vi "bats.parser.test.Single.SequencedUnitHeader.vi"() -> (3 "Passed":bool)   [LabVIEW 2022 SP3]
uses:
  pitch/AddOrder/AddOrderLong.Parameters.ctl
  pitch/ModifyOrder/ModifyOrderLong.Parameters.ctl
  <vilib>/Utility/error.llb/Trim Whitespace One-Sided.vi
  pitch/SequencedUnitHeader/SequencedUnitHeader.lvclass
  pitch/MessageBase/MessageBase.lvclass
  pitch/AddOrder/AddOrderLong.lvclass
  pitch/ModifyOrder/ModifyOrderLong.lvclass
panel:
  in  "ModifyOrderLong.Parameters":T1={"Time Offset"=0, "Order Id"="OD02", "Quantity"=50, "Price"=100.01, "Modify Flags"=1}
  in  "AddOrderLong.Parameters.2":T2={"Time Offset"=0, "Order Id"="OD02", "Quantity"=50, "Symbol"="AAPL", "Side Indicator"="S", "Price"=100.01}
  in  "AddOrderLong.Parameters.1":T2={"Time Offset"=1, "Order Id"="OD01", "Quantity"=10, "Symbol"="AAPL", "Side Indicator"="B", "Price"=100.05}
  out "# of Messages\nMatched?":bool[](array[boolean])
  out "Messages Matched?":bool[](array[boolean])=[TRUE]
  out "# of SeqHdUni Matched?":bool
  in  "Expected Results":cluster{string[]}[](array[cluster])=[{["OD01", "OD02", "OD02"]}]
  out "Results":cluster{string[]}[](array[cluster])
  out "Bytes.Out":u8[](array[numeric]) format="%.0x"
  out "Bytes.out (Visual)":u8[][](array[numeric]) format="%.0x"
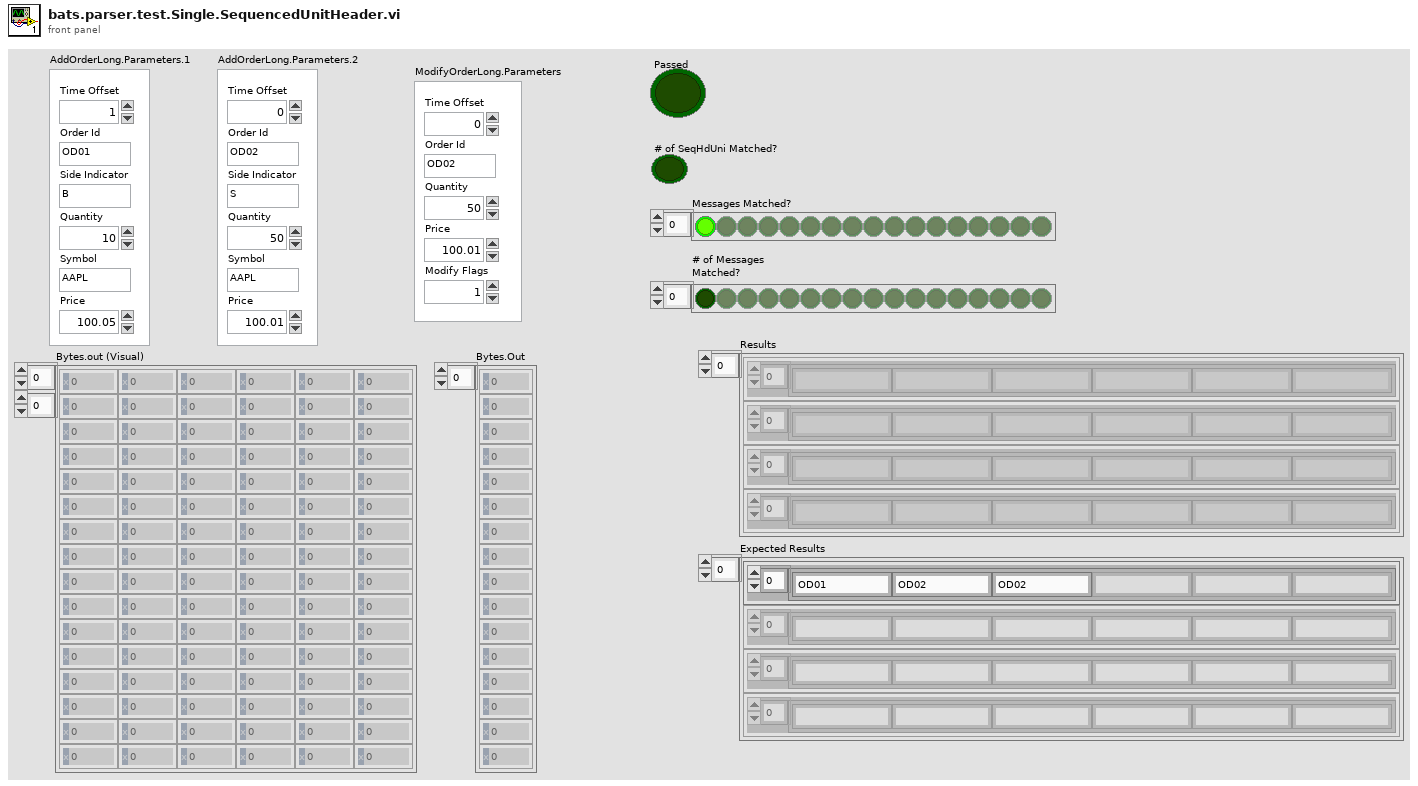
[diagram p1: front panel]
types:
  T1 = typedef "ModifyOrderLong.lvclass/ModifyOrderLong.Parameters.ctl" = cluster{"Time Offset":u32, "Order Id":string, "Quantity":u32, "Price":dbl, "Modify Flags":u8}
  T2 = typedef "AddOrderLong.lvclass/AddOrderLong.Parameters.ctl" = cluster{"Time Offset":u32, "Order Id":string, "Quantity":u32, "Symbol":string, "Side Indicator":string, "Price":dbl}
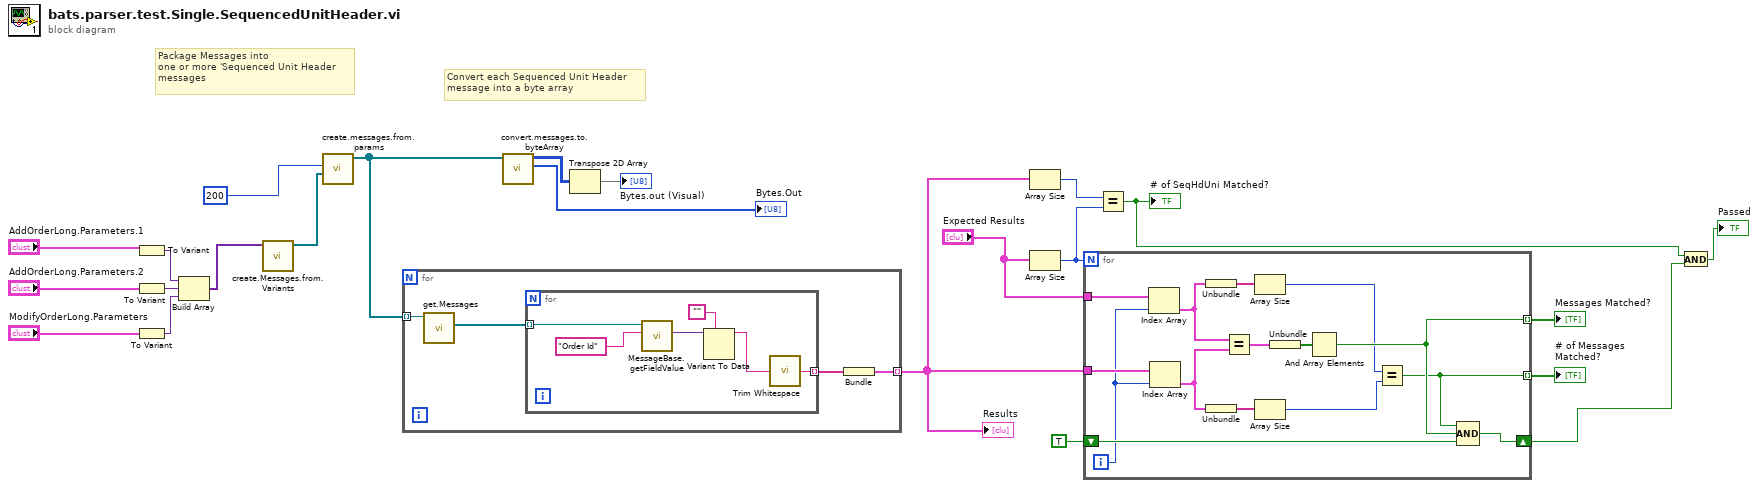
[diagram p0: block diagram]
diagram:
  # "Convert each Sequenced Unit Header\nmessage into a byte array"
  # "Package Messages into\none or more 'Sequenced Unit Header\nmessages"
  n1 = To Variant(anything="AddOrderLong.Parameters.1") -> (Variant=w5:variant)
  n2 = To Variant(anything="AddOrderLong.Parameters.2") -> (Variant=w4:variant)
  n3 = To Variant(anything="ModifyOrderLong.Parameters") -> (Variant=w3:variant)
  n4 = Build Array(w5, w4, w3) -> (w2:variant[])
  n5 = call "create.Messages.from.Variants.vi"("Messages.Variant"=w2) -> ("Messages"=w1:refnum<class "MessageBase.lvclass">[])  [unwired: 10 in]
  n6 = call "create.messages.from.params.vi"("Message.to.Create"=w1, "Max.Frame.Size"=u16 200) -> ("Messages.Out"=w19:refnum<class "SequencedUnitHeader.lvclass">[])  [unwired: 9 in]
  n7 = for {
    tunnel: w19 -> [w27] mode=indexing
    tunnel: [w24] -> w16 mode=indexing
    n8 = call-dynamic "get.Messages.vi"("SequencedUnitHeader in"=w27) -> ("Messages.Out"=w26:refnum<class "MessageBase.lvclass">[])  [unwired: 8 in, 2 out]
    n9 = for {
      tunnel: w26 -> [w31] mode=indexing
      tunnel: [w28] -> w25 mode=indexing
      n10 = call-dynamic "MessageBase.getFieldValue.vi"("FIeld.Name"="Order Id" ("Field.Name"), "MessageBase in"=w31) -> ("FieldValue"=w30:variant)  [unwired: 7 in, 2 out]
      n11 = Variant To Data(type="", Variant=w30) -> (data=w29:string)  [unwired: 1 in, 1 out]
      n12 = call <vilib>:"Trim Whitespace.vi"("string"=w29) -> ("trimmed string"=w28:string)  [unwired: 1 in]
    }
    n13 = Bundle(w25) -> (w24:cluster{string[]})  [unwired: 1 in]
  }
  "Results" <- w16
  n14 = call "convert.messages.to.byteArray.vi"("Messages.In"=w19) -> ("ByteArray.out"=→"Bytes.Out":u8[], "2D.ByteArray.out"=w22:u8[][])  [unwired: 9 in]
  n15 = Transpose 2D Array(2D array=w22) -> (transposed array=→"Bytes.out (Visual)":u8[][])
  n16 = Array Size(array=w16) -> (size(s)=w14:i32)
  n17 = Array Size(array="Expected Results") -> (size(s)=w15:i32)
  n18 = for {
    N: w15 -> [_]
    shift-right: [w47] -> w11
    shift-left: TRUE -> [w48]
    tunnel: w16 -> [w46]
    tunnel: "Expected Results" -> [w45]
    tunnel: [w41] -> w13 mode=indexing
    tunnel: [w34] -> w12 mode=indexing
    i -> [w44]
    n19 = Index Array(array=w45, index=w44) -> (element=w40:cluster{string[]})
    n20 = Index Array(array=w46, index=w44) -> (element=w39:cluster{string[]})
    n21 = Unbundle(w40) -> (w37:string[])
    n22 = Unbundle(w39) -> (w38:string[])
    n23 = Equal?(x=w40, y=w39) -> (x = y?=w43:cluster{bool[]})
    n24 = Array Size(array=w37) -> (size(s)=w36:i32)
    n25 = Array Size(array=w38) -> (size(s)=w35:i32)
    n26 = Unbundle(w43) -> (w42:bool[])
    n27 = And Array Elements(Boolean array=w42) -> (logical AND=w41:bool)
    n28 = Equal?(x=w36, y=w35) -> (x = y?=w34:bool)
    n29 = Compound Arithmetic op=AND(w34, w41, w48) -> (w47:bool)
  }
  "Messages Matched?" <- w13
  "# of Messages\nMatched?" <- w12
  n30 = Equal?(x=w14, y=w15) -> (x = y?=w10:bool)
  "# of SeqHdUni Matched?" <- w10
  n31 = And(x=w10, y=w11) -> (x .and. y?=→"Passed":bool)
